vi "PV ActiveLine - Example Read Pressure.vi"(7 "Baud Rate":u32(ring) items=["9600 (default)", "19200", "38400", "57600", "115200"], 8 "error in (no error)":errorcluster caption="Fehler (Eingang, kein Fehler)", 11 "input refnum":refnum<visa-resource-name> caption="Eingang (Referenz)") -> (0 "error out":errorcluster, 1 "Pressure Sensor 2":dbl format="%.3e", 2 "Pressure Sensor 1":dbl format="%.3e")   [LabVIEW 2013, in "PV ActiveLine.lvlib"]
doc: "This VI is an example of how to use the PV ActiveLine subVIs programmatically. This VI first initializes the instrument, takes measurements, then closes the instrument."
uses:
  PV ActiveLine.lvlib
panel:
  out "Status Sensor 2":i32(ring) items=["data OK", "underrange", "overrange", "sensor error", "sensor off", "no sensor", "ID error"]
  out "Status Sensor 1":i32(ring) items=["data OK", "underrange", "overrange", "sensor error", "sensor off", "no sensor", "ID error"]
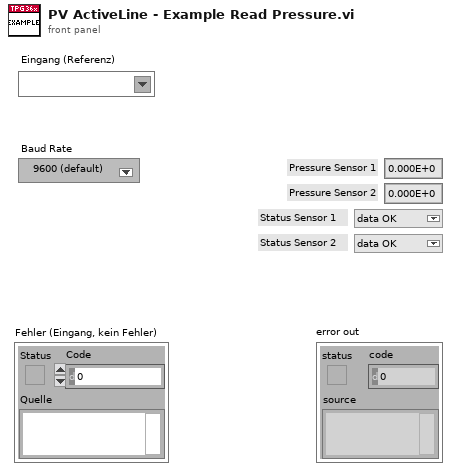
[diagram p1: front panel]
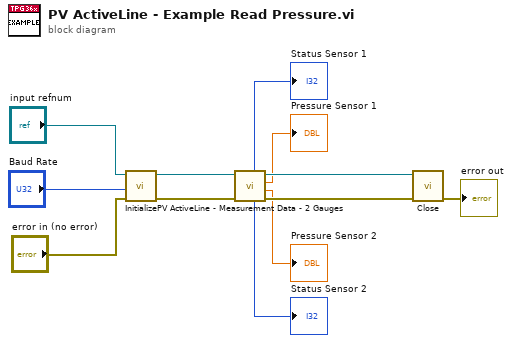
[diagram p0: block diagram]
diagram:
  n1 = call "Initialize.vi"("error in (no error)"="error in (no error)", "Baud Rate"="Baud Rate", "input refnum"="input refnum") -> ("Cluster (Ausgang)"=w7:errorcluster, "Referenz out"=w11:refnum<visa-resource-name>)  [unwired: 7 in]
  n2 = call "PV ActiveLine - Measurement Data - 2 Gauges.vi"("Fehler (Eingang)"=w7, "Referenz in"=w11) -> ("Cluster (Ausgang)"=w9:errorcluster, "Pressure Sensor 2"=→"Pressure Sensor 2":dbl, "Pressure Sensor 1"=→"Pressure Sensor 1":dbl, "Referenz out"=w10:refnum<visa-resource-name>, "Status Sensor 2"=→"Status Sensor 2":i32, "Status Sensor 1"=→"Status Sensor 1":i32)  [unwired: 4 in]
  n3 = call "Close.vi"("error in (no error)"=w9, "VISA resource name"=w10) -> ("error out"=→"error out":errorcluster)  [unwired: 9 in]
